vi "Allgemein.vi"(8 "Fehler (Eingang)":errorcluster) -> (0 "Fehler (Ausgang)":errorcluster)   [LabVIEW 2020, in "Allgemein.lvlib"]
uses:
  Allgemein.lvlib
  Stoermeldungen/Aktion Heizung Uebertemperatur.ctl
  Verwaltung/FGV OUT Aktionen.ctl
  Stoermeldungen/FGV Stoerungen Aktionen.ctl
  Verwaltung/FGV IN Aktionen.ctl
  Konfig-Dateien/FGV Betriebsdaten Aktionen.ctl
  Aktion FGV Zustandsbeleuchtung schalten.ctl
  Stoermeldungen/Stoermeldungen.lvlib
  Stickstoff Befuellung/Stickstoff Befuellung.lvlib
  Regler/Regler.lvlib
  Regler/FGV Daten Regler Aktionen.ctl
  Verwaltung/Verwaltung - cRIO.lvlib
  Konfig-Dateien/Konfig-Dateien.lvlib
  FGV FT-IR Kuehlung Aktionen.ctl
  Externe Stickstoff Befuellung/Externe Stickstoff Befuellung.lvlib
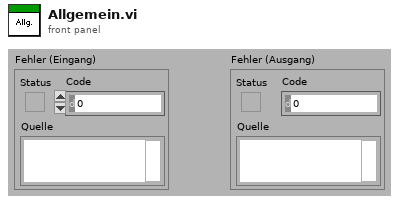
[diagram p1: front panel]
types:
  T1 = typedef "Konfig-Dateien.lvlib/FGV Betriebsdaten Aktionen.ctl" = enum16{"lesen", "Anlagengrenzw.", "PID Param.", "Sonstige", "Sensor Para."}
  T2 = typedef "Regler.lvlib/FGV Daten Regler Aktionen.ctl" = enum16{"lesen", "Out%", "Heizung EIN"}
  T3 = typedef "Anlagengrenzwerte.lvlib/Anlagen-Grenzwerte Anzeige.ctl" = cluster{"Eingangsdruck FT-IR:":T4, "Durchfluss FT-IR:":T4, "Durchfluss CalGas:":T4, "Druck Ausgang:":T4, "Druck Kalter Block:":T4, "Heizleitungen intern:":T4, "Heizleitung zu FT-IR:":T4, "Heizung Filterblock:":T4, "Heizung Pumpe:":T4, "Heizleitung Extern SP1:":T4, "Heizleitung Extern SP2:":T4, "FT-IR Heizung Messzelle:":T4, "Schaltschranktemperatur:":T4, "Gaskühler:":T4}
  T4 = typedef "Anlagengrenzwerte.lvlib/Anlagen-Parameter Anzeige.ctl" = cluster{"Sollwert":sgl, "Warn-Min":sgl, "Warn-Max":sgl, "Abschalt-Min":sgl, "Abschalt-Max":sgl, "Regler":u16}
  T5 = typedef "Erweiterte Konfig.lvlib/Sonstige Parameter.ctl" = cluster{"Lüfter langsam":sgl, "Lüfter schnell":sgl, "FT-IR Kühlung Soll":sgl, "FT-IR Kühlung Max":sgl, "Überwachung":T6, "Befüllung aktiv":T7, "Stickstoff Befüllzeit":sgl, "Befüllintervall":sgl, "Kalibrierwert FT-IR":sgl, "Offset Ausgang":sgl, "Offset FT-IR":sgl, "Offset Druck FT-IR":sgl, "Dichtheitstest Zeit":sgl, "Dichtheitstest Abfall":sgl, "Dichtheitstest Umfang":T8, "Offset Umgebung":sgl, "Max Taupunkt":sgl, "Pumpendrehzahl":sgl, "ext. Befüllung":T7, "Ext. Stickstoff Befüllzeit":sgl}
  T6 = typedef "Auswahlfeld.ctl" = u16
  T7 = typedef "LogKonfig.lvlib/Auswahlfeld aktiviert-deaktiviert.ctl" = u16
  T8 = typedef "Erweiterte Konfig.lvlib/Dichtheitstest Umfang.ctl" = u16
  T9 = cluster{"Output% 1":i16, "Output% 2":i16, "Output% 3":i16, "Output% 4":i16, "Output% 5":i16, "Output% 6":i16, "Output% 7":i16, "Output% 8":i16, "Output% 9":i16, "Output% 10":i16, "Output% 11":i16, "Output% 12":i16, "Output% 13":i16, "Output% 14":i16, "Output% 15":i16, "Output% 16":i16, "Output% 17":i16, "Output% 18":i16}
  T10 = typedef "Verwaltung - cRIO.lvlib/FGV OUT Aktionen.ctl" = enum16{"lesen", "ANA OUT", "DO 0-31", "DO 32-47"}
  T11 = typedef "Allgemein.lvlib/Aktion FGV Zustandsbeleuchtung schalten.ctl" = enum16{"lesen", "prüfen", "init", "Bit löschen", "ansteuern", "Aufheizphase"}
  T12 = typedef "Verwaltung - cRIO.lvlib/FGV IN Aktionen.ctl" = enum16{"lesen", "DI", "AI", "Fühler Br.", "TC", "Fühler Br. TC"}
  T13 = typedef "Stoermeldungen.lvlib/FGV Stoerungen Aktionen.ctl" = enum16{"lesen", "Störung aktiv?", "1-64", "65-128"}
  T14 = typedef "Stoermeldungen.lvlib/Aktion Heizung Uebertemperatur.ctl" = enum16{"lesen", "prüfen", "rücksetzen"}
  T15 = typedef "Allgemein.lvlib/FGV FT-IR Kuehlung Aktionen.ctl" = enum16{"lesen", "Kühlung?"}
  T16 = typedef "Verwaltung - cRIO.lvlib/Digital Eingaenge 0-15.ctl" = cluster{"I0: N2 Nachf. FT-IR voll":bool, "I1: N2 Nachf. Vorrat leer":bool, "I2: (Klimaanlage eingeschaltet)":bool, "I3: (Klimaanlage Störung)":bool, "I4: Trigger Eingang (Messdaten sp.)":bool, "I5: Reserve":bool, "I6: Reserve":bool, "I7: Reserve":bool, "I8: Druckschalter Versorgung ok":bool, "I9: Reserve":bool, "I10: Reserve":bool, "I11: Reserve":bool, "I12: Drucksch. N2 Versorgung":bool, "I13: Reserve":bool, "I14: Drucksch. N2 Optikbox":bool, "I15: (Füllstand Kondensatbehälter)":bool}
  T17 = typedef "Verwaltung - cRIO.lvlib/TC Eingaenge.ctl" = cluster{"TC0: Reserve":sgl, "TC1: HL zu FT-IR":sgl, "TC2: HL Extern SP1":sgl, "TC3: HL Extern SP2":sgl, "TC4: Reserve":sgl, "TC5: Reserve":sgl, "TC6: Reserve":sgl, "TC7: Reserve":sgl, "TC8: FT-IR":sgl, "TC9: Reserve":sgl, "TC10: Schaltschrank":sgl, "TC11: Umgebung":sgl}
  T18 = typedef "Verwaltung - cRIO.lvlib/Digital Ausgaenge 32-63.ctl" = cluster{"O32: Messgaspumpe EIN":bool, "O33: (Umgebungsluftpumpe)":bool, "O34: (Kondensatpumpe GK)":bool, "O35: Klima/Lüfter EIN":bool, "O36: Versorgung Heizungen":bool, "O37: Versorgung Heizungen":bool, "O38: (Gaskühler EIN (Freigabe))":bool, "O39: Störung FAS LP":bool, "O40: (Heizung Filterblock)":bool, "O41: Heizung HL zu FT-IR":bool, "O42: Heizung HL Extern SP1":bool, "O43: Heizung HL Extern SP2":bool, "O44: Heizung Reserve":bool, "O45: Heizung Reserve":bool, "O46: Statusbeleuchtung grün":bool, "O47: Statusbeleuchtung rot":bool}
  T19 = typedef "Verwaltung - cRIO.lvlib/Digital Ausgaenge 0-31.ctl" = cluster{"O0: Druckluft Versorgung":bool, "O1: CG 1 (FB Eingang 1)":bool, "O2: CG 2 (Kühlung FT-IR EIN)":bool, "O3: CG 3 (FB Bypass)":bool, "O4: CG 4 (FB CalGas)":bool, "O5: CG 5 (FB spülen/UL)":bool, "O6: CG 6 (FB zum FT-IR)":bool, "O7: CG 7 (FB zum FID)":bool, "O8: CG 8 (FB Reserve)":bool, "O9: (FB Reserve)":bool, "O10: (FB Umgebungsluft FID)":bool, "O11: (FB zum Gaskühler)":bool, "O12: FB Stickstoff zu FT-IR":bool, "O13: Optikbox FT-IR spülen":bool, "O14: (Purifier deaktivieren)":bool, "O15: (Umschaltung Purifier/Stickstoff)":bool, "O16: N2 Einblasung":bool, "O17: LSP LN2 Nachfüllung":bool, "O18: (Reserve)":bool, "O19: (Pumpe Eingang1)":bool, "O20: (Pumpe Eingang2)":bool, "O21: (Pumpe Spülen1)":bool, "O22: (Pumpe Spülen2)":bool, "O23: (Reserve)":bool, "O24: CalGas 1":bool, "O25: CalGas 2":bool, "O26: CG 3-8 (CalGas 3)":bool, "O27: Stickstoff aufschalten":bool, "O28: CG zu PNS":bool, "O29: FTIR Standby Spülung":bool, "O30: CG zu Entnahme(T90)":bool, "O31: (Purifier regenerieren)":bool}
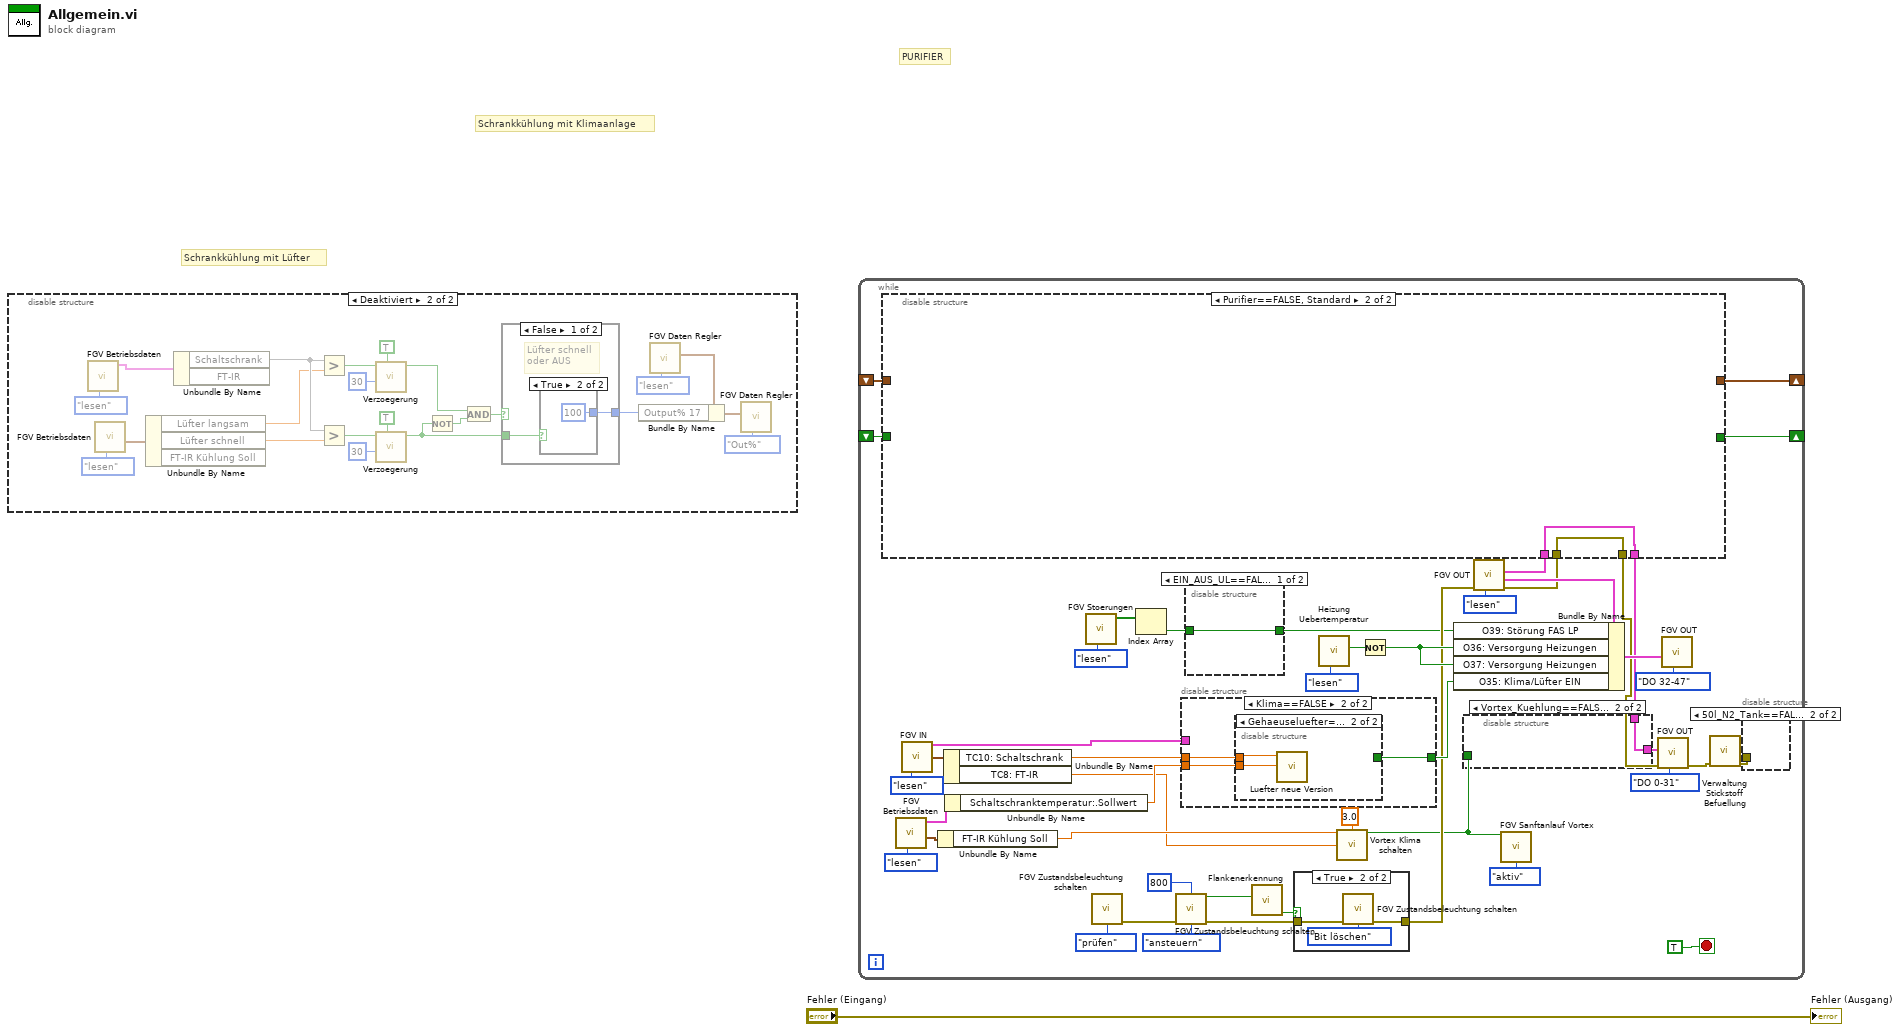
[diagram p0: block diagram]
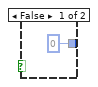
[diagram p3: hidden frame]
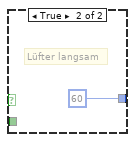
[diagram p4: hidden frame]
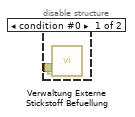
[diagram p5: hidden frame]
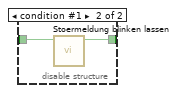
[diagram p6: hidden frame]
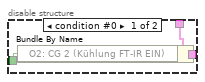
[diagram p7: hidden frame]
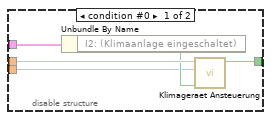
[diagram p9: hidden frame]
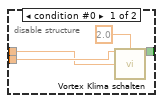
[diagram p10: hidden frame]
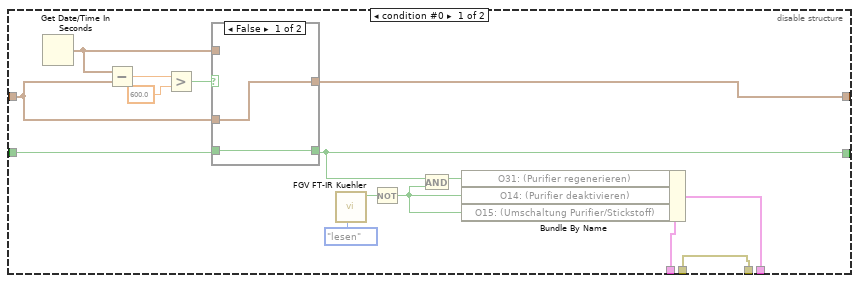
[diagram p11: hidden frame]
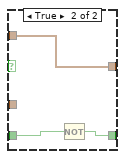
[diagram p12: hidden frame]
diagram:
  # "PURIFIER"
  # "Schrankkühlung mit Klimaanlage"
  # "Schrankkühlung mit Lüfter"
  n1 = disable-structure shown="Deaktiviert" {
    frame Enabled {
    }
    frame Disabled {
      n2 = call "FGV Betriebsdaten.vi"("Aktionen"=FGV_Betriebsdaten_Aktionen."lesen") -> ("Anlagen-Grenzwerte"=w25:T3)  [unwired: 7 in, 3 out]
      n3 = call "FGV Betriebsdaten.vi"("Aktionen"=FGV_Betriebsdaten_Aktionen."lesen") -> ("Sonstige"=w2:T5)  [unwired: 7 in, 3 out]
      n4 = Unbundle By Name(w2) -> ("Lüfter langsam"=w9:sgl, "Lüfter schnell"=w11:sgl, "FT-IR Kühlung Soll"=w23:sgl)
      n5 = Unbundle By Name(w25) -> ("Schaltschrank"=w10, "FT-IR"=w22)
      n6 = Greater?(x=w10, y=w9) -> (0:w14:bool)
      n7 = Greater?(x=w10, y=w11) -> (0:w16:bool)
      n8 = call "Verzoegerung.vi"("Abfallverzögerung?"=TRUE, "sec"=u16 30, "Startsignal"=w14) -> ("Zeit abgelaufen?"=w15:bool)  [unwired: 7 in, 1 out]
      n9 = call "Verzoegerung.vi"("Abfallverzögerung?"=TRUE, "sec"=u16 30, "Startsignal"=w16) -> ("Zeit abgelaufen?"=w17:bool)  [unwired: 7 in, 1 out]
      n10 = Not(x=w17) -> (.not. x?=w12:bool)
      n11 = And(x=w15, y=w12) -> (x .and. y?=w13:bool)
      n12 = case shown="False" w13 {
        tunnel: [w27 i16 60 ("Output% 12")] -> w4
        tunnel: w17 -> [w26 _]
        frame False {
          # "Lüfter schnell\noder AUS"
          n13 = case shown="True" w26 {
            tunnel: [i16 0 ("Output% 12") i16 100 ("Output% 12")] -> w27
            frame False {
            }
            frame True {
            }
          }
        }
        frame True {
          # "Lüfter langsam"
        }
      }
      n14 = call "FGV Daten Regler.vi"("Aktionen"=FGV_Daten_Regler_Aktionen."lesen") -> ("PID - OUT%"=w7:T9)  [unwired: 9 in, 1 out]
      n15 = Bundle By Name(cluster=w7, "Output% 17"=w4) -> (w5:T9)
      n16 = call "FGV Daten Regler.vi"("Aktionen"=FGV_Daten_Regler_Aktionen."Out%", "PID - OUT%"=w5) -> ()  [unwired: 8 in, 2 out]
    }
  }
  n17 = while {
    shift-right: [w69] -> _
    shift-left: _ -> [w68]
    shift-right: [w66] -> _
    shift-left: _ -> [w67]
    stop <- TRUE stop-if-true
    n18 = call "FGV Betriebsdaten.vi"("Aktionen"=FGV_Betriebsdaten_Aktionen."lesen") -> ("Sonstige"=w43:T5, "Anlagen-Grenzwerte"=w60:T3)  [unwired: 7 in, 2 out]
    n19 = call "FGV IN.vi"("Aktion"=FGV_IN_Aktionen."lesen") -> ("DI"=w63:T16, "TC Eingänge"=w62:T17)  [unwired: 10 in, 3 out]
    n20 = Unbundle By Name(w43) -> ("FT-IR Kühlung Soll"=w41:sgl)
    n21 = Unbundle By Name(w62) -> ("TC10: Schaltschrank"=w65:sgl, "TC8: FT-IR"=w40:sgl)
    n22 = Unbundle By Name(w60) -> ("Schaltschranktemperatur:.Sollwert"=w59:sgl)
    n23 = call "FGV Stoerungen.vi"("Aktionen"=FGV_Stoerungen_Aktionen."lesen") -> ("Störung aktiv?"=w47:bool[])  [unwired: 8 in, 2 out]
    n24 = call "FGV Zustandsbeleuchtung schalten.vi"("Aktion"=Aktion_FGV_Zustandsbeleuchtung_schalten."prüfen") -> ("error out"=w53:errorcluster)  [unwired: 13 in, 1 out]
    n25 = Index Array(array=w47) -> (element=w31:bool)  [unwired: 1 in]
    n26 = call "FGV Zustandsbeleuchtung schalten.vi"("Blinkgeschwindigkeit in ms"=800, "error in (no error)"=w53, "Aktion"=Aktion_FGV_Zustandsbeleuchtung_schalten."ansteuern") -> ("Aufheizphase"=w51:bool, "error out"=w49:errorcluster)  [unwired: 11 in]
    n27 = disable-structure shown="Klima==FALSE" {
      disable-tunnel: w65 -> [w93 w95]
      disable-tunnel: w63 -> [w91 _]
      disable-tunnel: w59 -> [w90 w96]
      disable-tunnel: [w89 w94] -> w58
      frame condition #0 {
        n28 = Unbundle By Name(w91) -> ("I2: (Klimaanlage eingeschaltet)"=w92:bool)
        n29 = call "Klimageraet Ansteuerung.vi"("Service aktiv"=w92, "Einschalten ab"=w90, "Schaltschranktemperatur"=w93) -> ("Klimagerät EIN"=w89:bool)  [unwired: 8 in]
      }
      frame condition #1 (active) {
        n30 = disable-structure shown="Gehaeuseluefter==TRUE" {
          disable-tunnel: w96 -> [w100 w102]
          disable-tunnel: w95 -> [w99 w101]
          disable-tunnel: [w97 _] -> w94
          frame condition #0 {
            n31 = call "Vortex Klima schalten.vi"("SOLL Temperatur"=w100, "Delta T"=sgl 2.0, "IST Temperatur"=w99) -> ("Ansteuerung"=w97:bool)  [unwired: 11 in, 1 out]
          }
          frame condition #1 (active) {
            n32 = call "Luefter neue Version.vi"("Lüfter"=w102, "Schaltschranktemp."=w101) -> ()  [unwired: 10 in]
          }
        }
      }
    }
    n33 = disable-structure shown="EIN_AUS_UL==FALSE, Standard" {
      disable-tunnel: [w78 w79] -> w32
      disable-tunnel: w31 -> [w78 w80]
      frame condition #0 (active) {
      }
      frame condition #1 {
        n34 = call "Stoermeldung blinken lassen.vi"("Fehler steht an"=w80) -> ("Blinken"=w79:bool)  [unwired: 9 in, 1 out]
      }
    }
    n35 = call "Flankenerkennung.vi"("Eingang"=w51) -> ("Fallende Flanke"=w50:bool)  [unwired: 9 in, 1 out]
    n36 = case shown="True" w50 {
      tunnel: w49 -> [w85 w87]
      tunnel: [w85 w86] -> w48
      frame False {
      }
      frame True {
        n37 = call "FGV Zustandsbeleuchtung schalten.vi"("error in (no error)"=w87, "Aktion"=Aktion_FGV_Zustandsbeleuchtung_schalten."Bit löschen") -> ("error out"=w86:errorcluster)  [unwired: 12 in, 1 out]
      }
    }
    n38 = call "Heizung Uebertemperatur.vi"("Aktionen"=Aktion_Heizung_Uebertemperatur."lesen") -> ("Heizung Übertemperatur"=w75:bool)  [unwired: 9 in, 1 out]
    n39 = call "Vortex Klima schalten.vi"("SOLL Temperatur"=w41, "Delta T"=sgl 3.0, "IST Temperatur"=w40) -> ("Ansteuerung"=w37:bool)  [unwired: 11 in, 1 out]
    n40 = Not(x=w75) -> (.not. x?=w70:bool)
    n41 = call "FGV OUT.vi"("Aktion"=FGV_OUT_Aktionen."lesen", "error in (no error)"=w48) -> ("error out"=w35:errorcluster, "DO 32-63"=w56:T18, "DO 0-31"=w45:T19)  [unwired: 6 in, 1 out]
    n42 = disable-structure shown="Purifier==FALSE, Standard" {
      disable-tunnel: w45 -> [w108 w124]
      disable-tunnel: [w117 _] -> w69
      disable-tunnel: w68 -> [w116 _]
      disable-tunnel: w67 -> [w115 _]
      disable-tunnel: [w110 _] -> w66
      disable-tunnel: [w104 w124] -> w36
      disable-tunnel: w35 -> [w103 w123]
      disable-tunnel: [w103 w123] -> w34
      frame condition #0 {
        n43 = Get Date/Time In Seconds() -> (seconds since 1Jan1904=w114:timestamp)
        n44 = Subtract(x=w114, y=w116) -> (x-y=w111:dbl)
        n45 = Greater?(x=w111, y=600.0) -> (0:w113:bool)
        n46 = case shown="False" w113 {
          tunnel: w116 -> [w119 _]
          tunnel: w114 -> [_ w122]
          tunnel: [w119 w122] -> w117
          tunnel: w115 -> [w118 w121]
          tunnel: [w118 w120] -> w110
          frame False {
          }
          frame True {
            n47 = Not(x=w121) -> (.not. x?=w120:bool)
          }
        }
        n48 = call "FGV FT-IR Kuehler.vi"("Aktionen"=FGV_FT-IR_Kuehlung_Aktionen."lesen") -> ("mit GN2 spülen"=w106:bool)  [unwired: 6 in, 4 out]
        n49 = Not(x=w106) -> (.not. x?=w105:bool)
        n50 = And(x=w110, y=w105) -> (x .and. y?=w107:bool)
        n51 = Bundle By Name(cluster=w108, "O31: (Purifier regenerieren)"=w107, "O14: (Purifier deaktivieren)"=w105, "O15: (Umschaltung Purifier/Stickstoff)"=w105) -> (w104:T19)
      }
      frame condition #1 (active) {
      }
    }
    n52 = Bundle By Name(cluster=w56, "O39: Störung FAS LP"=w32, "O36: Versorgung Heizungen"=w70, "O37: Versorgung Heizungen"=w70, "O35: Klima/Lüfter EIN"=w58) -> (w72:T18)
    n53 = disable-structure shown="Vortex_Kuehlung==FALSE" {
      disable-tunnel: w36 -> [w83 w84]
      disable-tunnel: [w82 w84] -> w44
      disable-tunnel: w37 -> [w81 _]
      frame condition #0 {
        n54 = Bundle By Name(cluster=w83, "O2: CG 2 (Kühlung FT-IR EIN)"=w81) -> (w82:T19)
      }
      frame condition #1 (active) {
      }
    }
    n55 = call "FGV Sanftanlauf Vortex.vi"("Flanke"=w37, "Aktion"=enum16{"init", "aktiv"}."aktiv") -> ()  [unwired: 12 in, 2 out]
    n56 = call "FGV OUT.vi"("Aktion"=FGV_OUT_Aktionen."DO 0-31", "error in (no error)"=w34, "DO 0-31"=w44) -> ("error out"=w39:errorcluster)  [unwired: 5 in, 3 out]
    n57 = call "FGV OUT.vi"("Aktion"=FGV_OUT_Aktionen."DO 32-47", "DO 32-63"=w72) -> ()  [unwired: 6 in, 4 out]
    n58 = call "Verwaltung Stickstoff Befuellung.vi"("Fehler (Eingang)"=w39) -> ("Fehler (Ausgang)"=w33:errorcluster)  [unwired: 10 in]
    n59 = disable-structure shown="50l_N2_Tank==FALSE, Standard" {
      disable-tunnel: w33 -> [w77 _]
      frame condition #0 {
        n60 = call "Verwaltung Externe Stickstoff Befuellung.vi"("Fehler (Eingang)"=w77) -> ()  [unwired: 10 in, 1 out]
      }
      frame condition #1 (active) {
      }
    }
  }
  "Fehler (Ausgang)" <- "Fehler (Eingang)"
